vi "write status log.vi"(8 "error in":errorcluster, 9 "Notes":string, 10 "Counter":i32, 11 "operation":string) -> (0 "error out":errorcluster)   [LabVIEW 2019, in "RemoteControl.ZMQ.lvlib" / "RemoteControl.ZMQ.lvclass"]
uses:
  RemoteControl.ZMQ.lvclass
  <vilib>/Utility/sysdir.llb/System Directory Type.ctl
  <vilib>/Utility/file.llb/Write Delimited Spreadsheet (string).vi
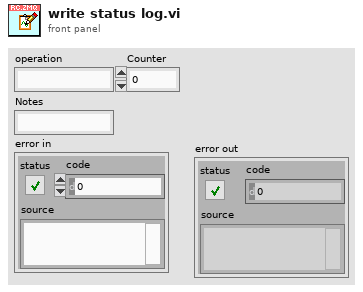
[diagram p1: front panel]
types:
  T1 = typedef "System Directory Type.ctl" = i32
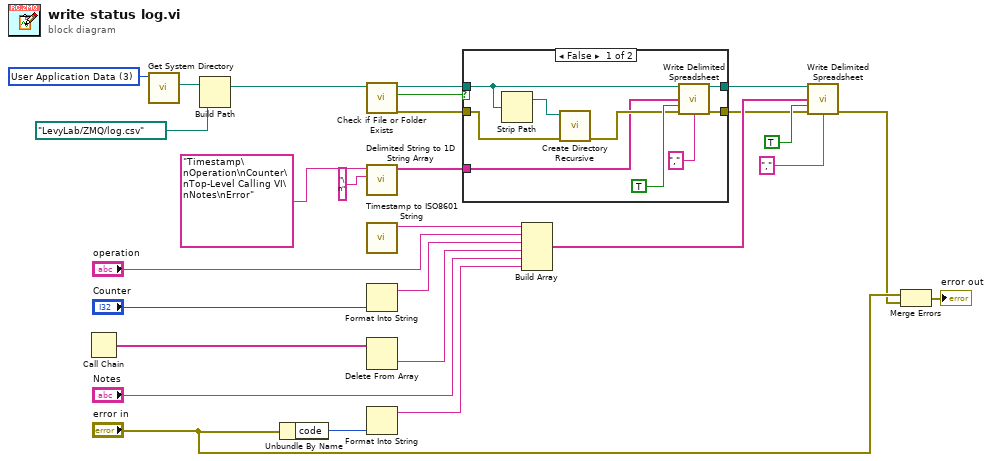
[diagram p0: block diagram]
diagram:
  w26 = T1 3 items=["User Home"=0, "User Desktop"=1, "User Documents"=2, "User Application Data"=3, "User Preferences"=4, "User Temporary"=5, "Public Documents"=6, "Public Application Data"=7, "Public Preferences"=8, "Public Cache"=13, "System Core Libraries"=9, "System Installed Libraries"=10, "Application Files"=11, "Boot Volume Root"=12] ("system directory type")
  n1 = Call Chain() -> (call chain=w1:string[])
  n2 = call <vilib>:"Get System Directory.vi"("system directory type"=w26) -> ("system directory"=w25:path)  [unwired: 10 in]
  n3 = Build Path(base path=w25, name or relative path=path "LevyLab/ZMQ/log.csv") -> (appended path=w23:path)
  n4 = Unbundle By Name("error in") -> ("code"=w10:i32)
  n5 = call <vilib>:"Check if File or Folder Exists.vi"("path"=w23) -> ("error out"=w11:errorcluster, "file or folder exists?"=w21:bool, "dup path"=w22:path)  [unwired: 8 in]
  n6 = call <vilib>:"Delimited String to 1D String Array.vi"("delimiter"="\n", "delimited string"="Timestamp\nOperation\nCounter\nTop-Level Calling VI\nNotes\nError") -> ("string array"=w24:string[])  [unwired: 9 in]
  n7 = call <vilib>:"Timestamp to ISO8601 String.vi"() -> ("ISO8601 String"=w20:string)  [unwired: 11 in]
  n8 = Format Into String("Counter") -> (resulting string=w17:string)  [unwired: 3 in, 1 out]
  n9 = Delete From Array(array=w1) -> (deleted portion=w2:string)  [unwired: 2 in, 1 out]
  n10 = Format Into String(w10) -> (resulting string=w9:string)  [unwired: 3 in, 1 out]
  n11 = case shown="False" w21 {
    tunnel: w24 -> [w30 _]
    tunnel: w22 -> [w33 w37]
    tunnel: [w35 w37] -> w14
    tunnel: [w34 w38] -> w12
    tunnel: w11 -> [w28 w38]
    frame False {
      n12 = Strip Path(path=w33) -> (stripped path=w32:path)  [unwired: 1 out]
      n13 = call <vilib>:"Create Directory Recursive.vi"("error in (no error)"=w28, "directory"=w32) -> ("error out"=w31:errorcluster)  [unwired: 3 in, 2 out]
      n14 = call-poly <vilib>:"Write Delimited Spreadsheet.vi"("file path (dialog if empty)"=w33, "1D data"=w30, "append to file? (new file:F)"=TRUE, "error in (no error)"=w31, "delimiter (\\t)"="," ("delimiter (\\t)")) -> ("new file path (Not A Path if cancelled)"=w35:path, "error out"=w34:errorcluster)  [unwired: 9 in]
    }
    frame True {
    }
  }
  n15 = Build Array(w20, "operation", w17, w2, "Notes", w9) -> (w13:string[])
  n16 = call-poly <vilib>:"Write Delimited Spreadsheet.vi"("file path (dialog if empty)"=w14, "1D data"=w13, "append to file? (new file:F)"=TRUE, "error in (no error)"=w12, "delimiter (\\t)"="," ("delimiter (\\t)")) -> ("error out"=w5:errorcluster)  [unwired: 9 in, 1 out]
  n17 = Merge Errors("error in", w5) -> (→"error out":errorcluster)
